vi "DataCluster.vi"() -> ()   [LabVIEW 2024]
uses:
  controls/#typedef_Waveform_Type.ctl
panel:
  in  "Main Data Cluster":T2
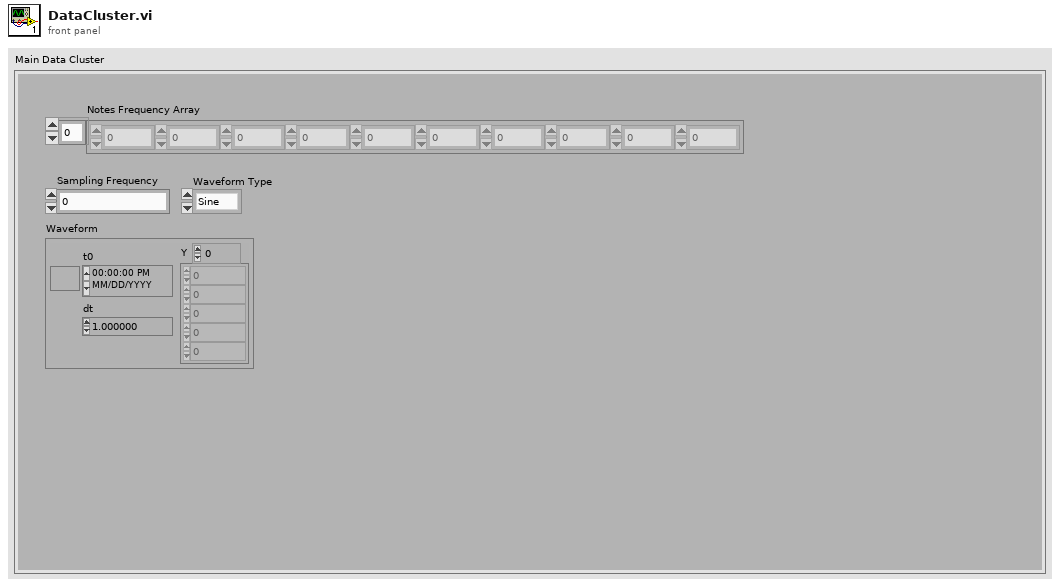
[diagram p1: front panel]
types:
  T1 = typedef "#typedef_Waveform_Type.ctl" = enum16{"Sine", "Saw", "Square", "Noise"}
  T2 = cluster{"Notes Frequency Array":dbl[], "Waveform":waveform(dbl), "Sampling Frequency":dbl, "Waveform Type":T1}
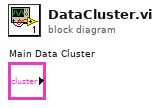
[diagram p0: block diagram]
diagram:
